vi "AlGaAs_SL_v07.vi"(2 "Debug Mode":bool, 3 "Elapsed Time(s)":dbl, 4 "State":enum16{"Edit", "Start", "Run", "End", "Idle"}(ring), 5 "Argument List In":string[](array[string])) -> (0 "Status Out":string, 1 "Argument List Out":string[](array[string]))   [LabVIEW 2011]
panel:
  out "tTotal(s) 2":dbl
  out "is_OK":bool
  out "tTotal(s)":dbl
  out "Do wait 2":bool
  out "Do wait 1":bool
  in  "Tab Control":enum32{"Step 1", "Step 2"}(tab)
  in  "run Ga 1":bool caption="run Ga"
  in  "run Al 1":bool=TRUE caption="run Al"
  in  "Al flow 1":dbl caption="Al flow(0-100sccm)" format="%.1f"
  in  "tFlow 1":dbl caption="tFlow(s)"
  in  "tWait(s) 1":dbl caption="tWait(s)"
  in  "Ga flow 1":dbl caption="Ga flow(0-10sccm)" format="%.3f"
  in  "fGa dilution 1":dbl caption="fGa dilution(>=1)"
  in  "run Ga 2":bool=TRUE caption="run Ga"
  in  "run Al 2":bool caption="run Al"
  in  "fGa 2":dbl caption="fGa dilution(>=1)"
  in  "Al flow 2":dbl caption="Al flow (0-100sccm)" format="%.1f"
  in  "Ga flow 2":dbl caption="Ga flow (0-10sccm)" format="%.3f"
  in  "tFlow 2":dbl caption="tFlow(s)"
  in  "tWait 2":dbl caption="tWait(s)"
  out "tphase(s)":dbl[](array[numeric])
  out "nstep":dbl
  out "phase":i32
  out "is_done":bool
  in  "nPeriods":dbl
  out "tPeriod(s)":dbl
  in  "Cancel":bool
  in  "OK":bool
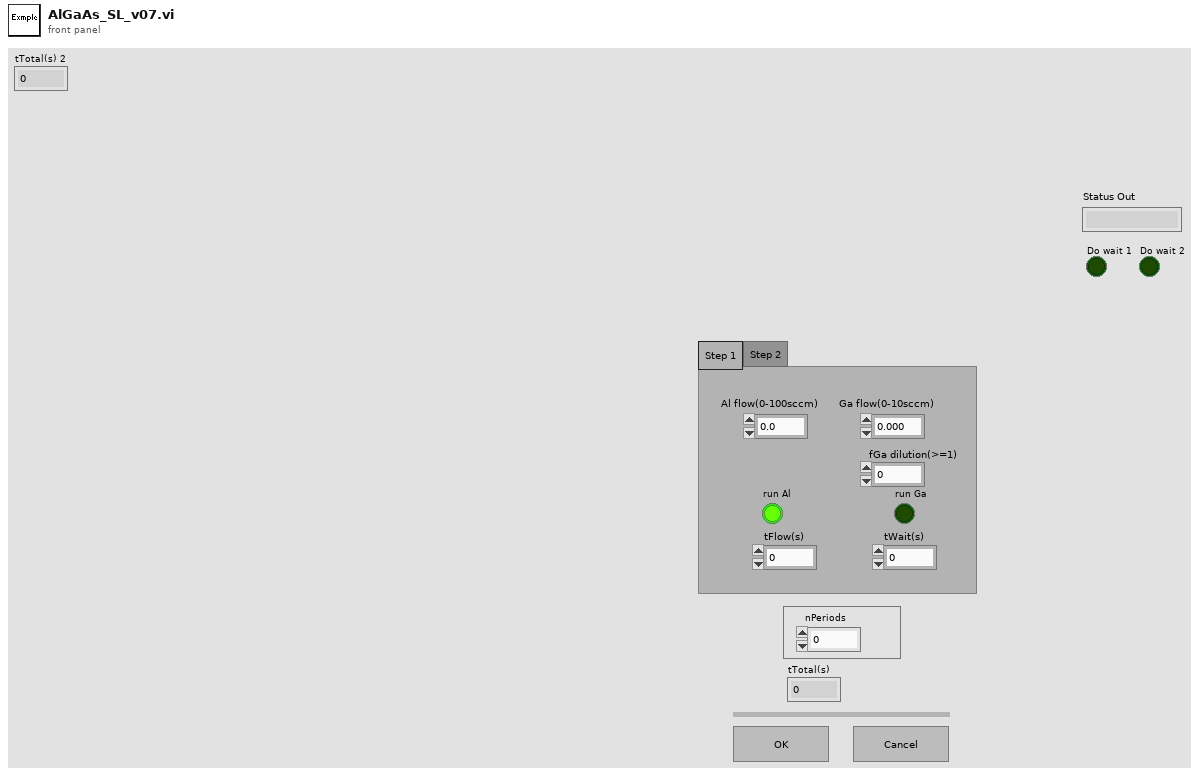
[diagram p1: front panel]
types:
  T1 = enum16{"Discrete", "Continuous", "Instantaneous"}
  T2 = enum32{"Invalid", "Default", "Floating", "Floating/Auto-Hide", "Modal"}
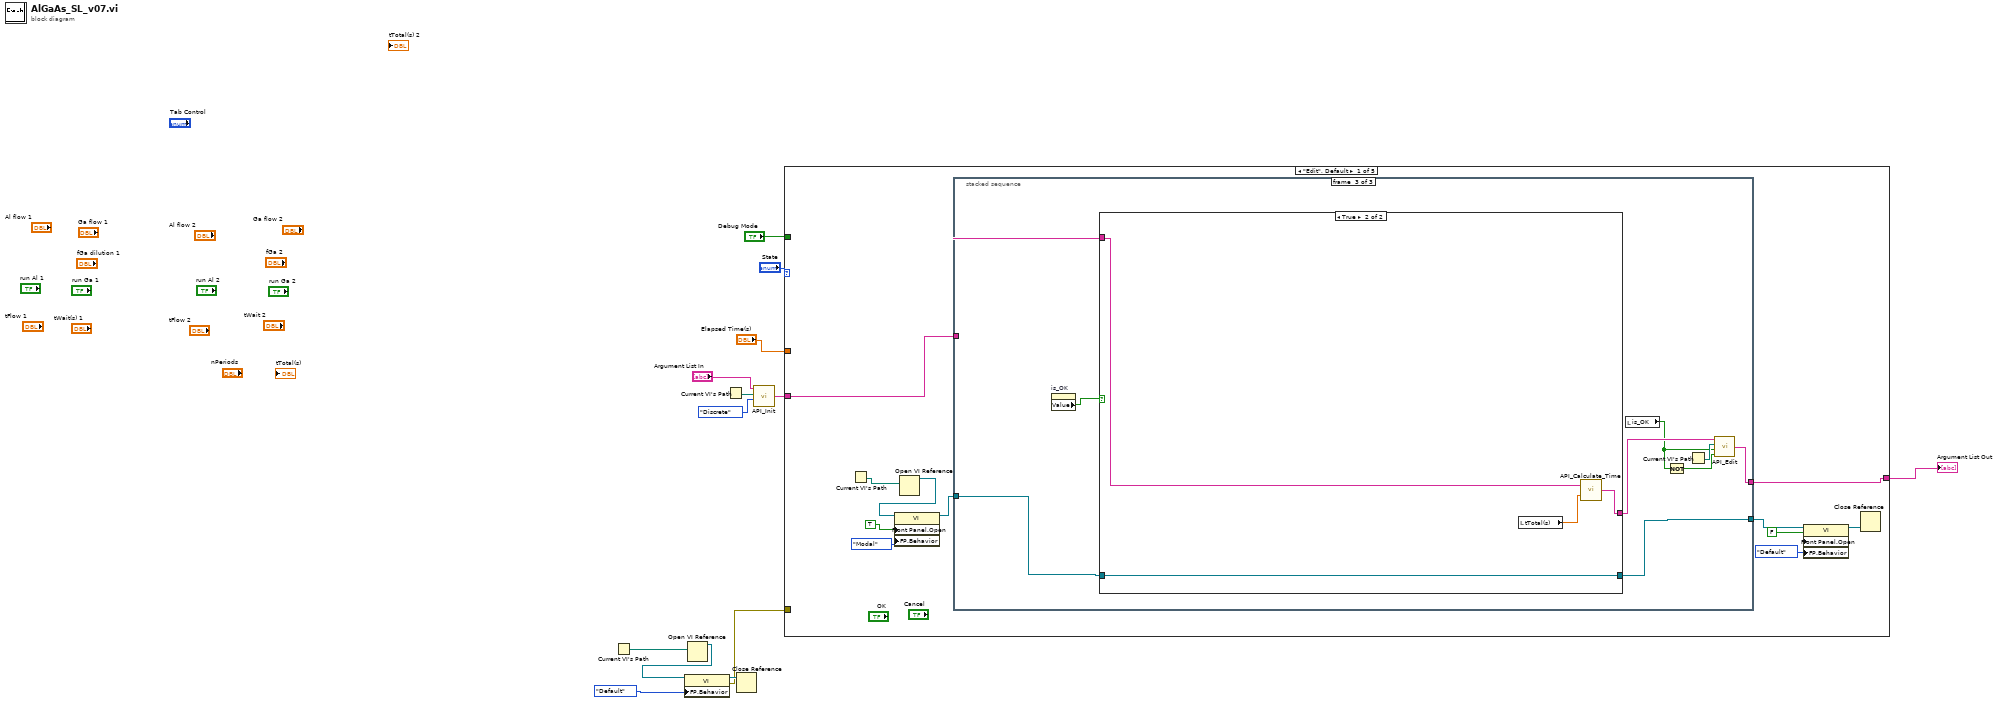
[diagram p0: block diagram]
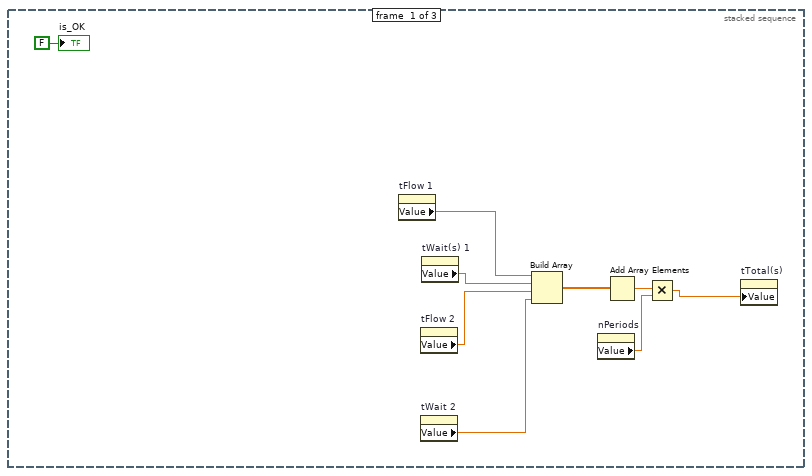
[diagram p2: hidden frame]
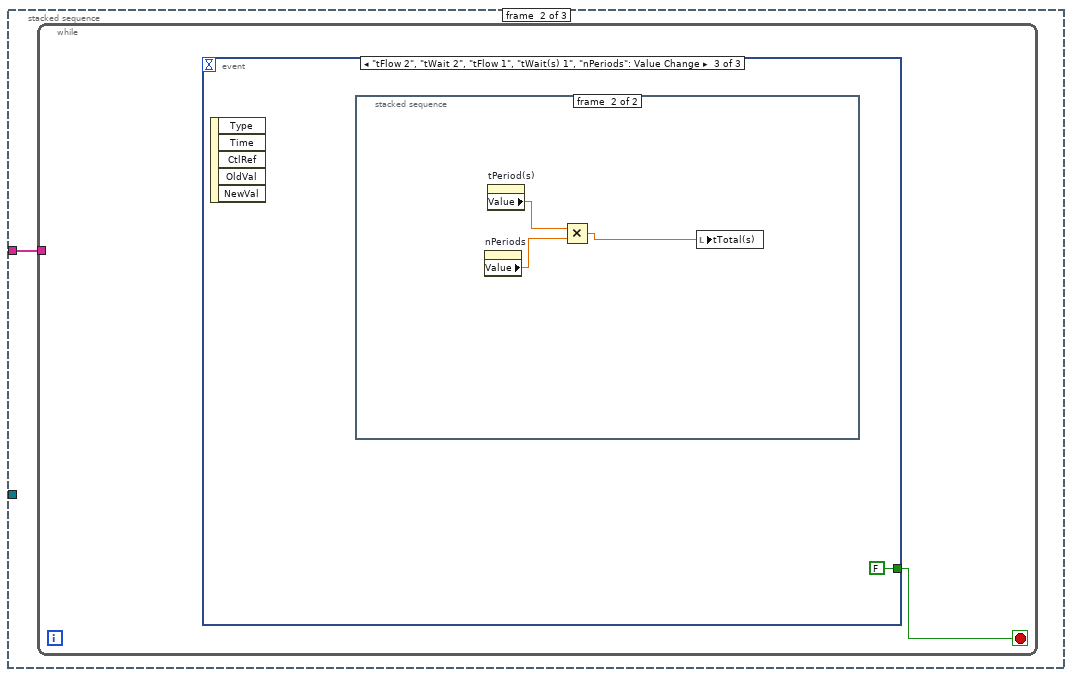
[diagram p3: hidden frame]
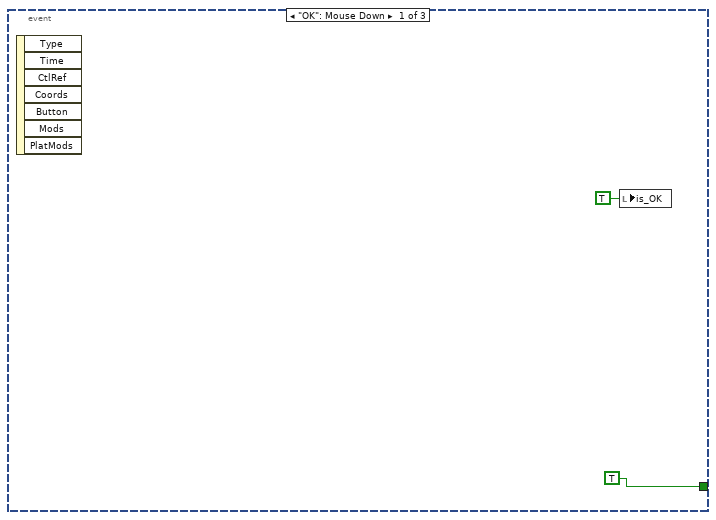
[diagram p4: hidden frame]
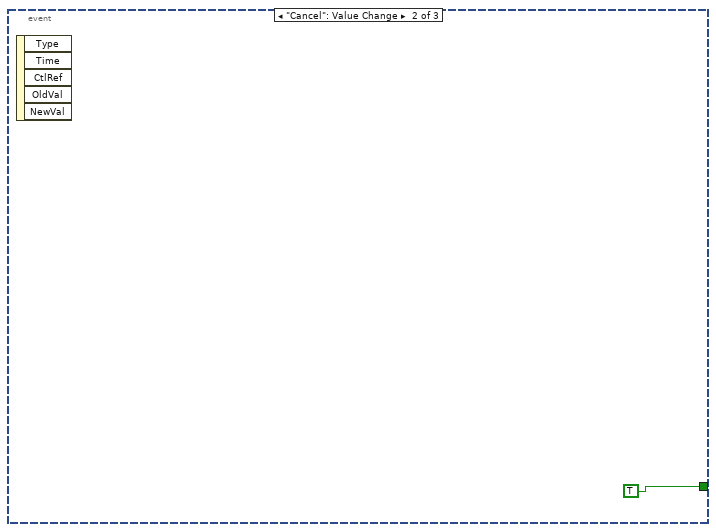
[diagram p5: hidden frame]
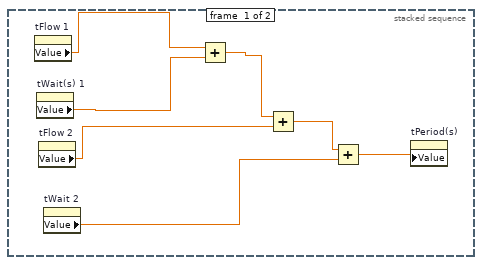
[diagram p6: hidden frame]
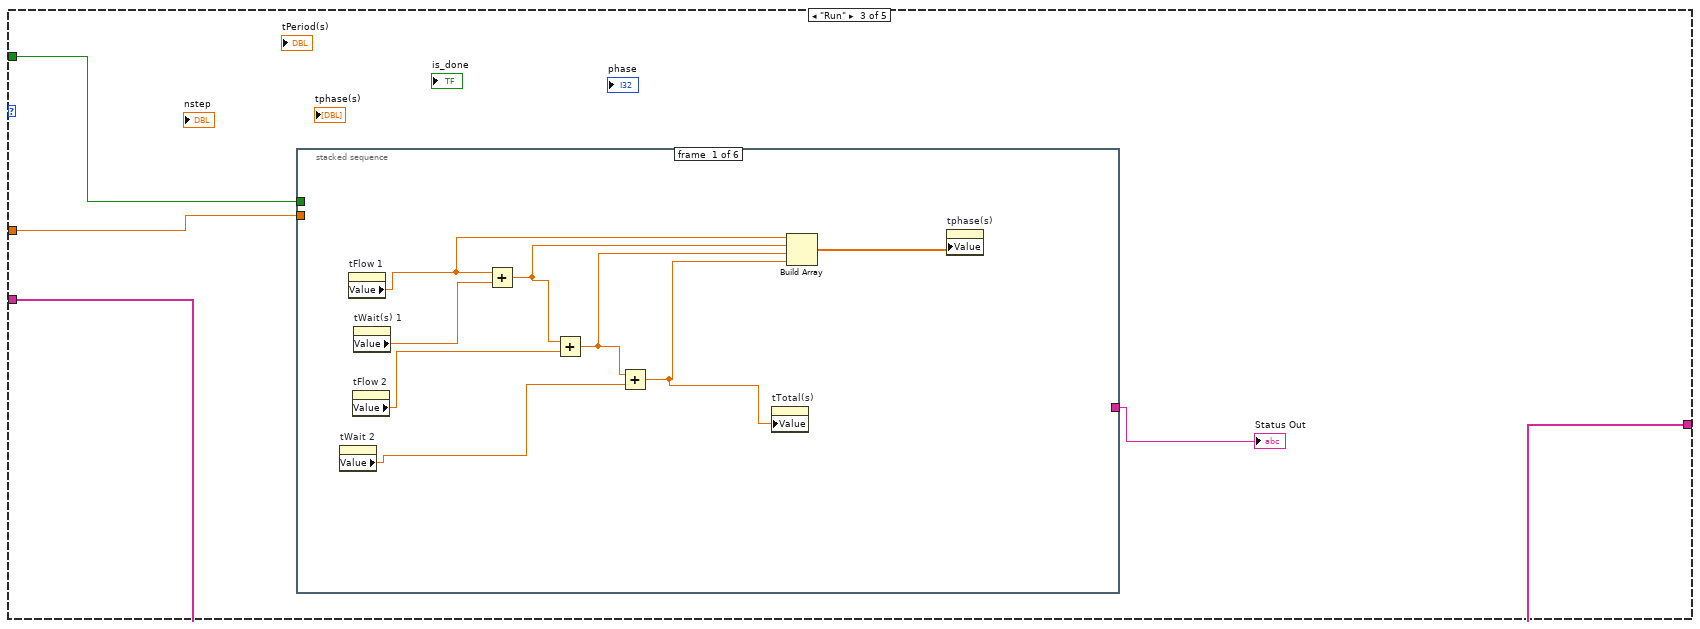
[diagram p9: hidden frame]
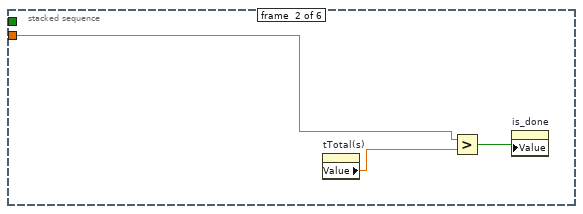
[diagram p10: hidden frame]
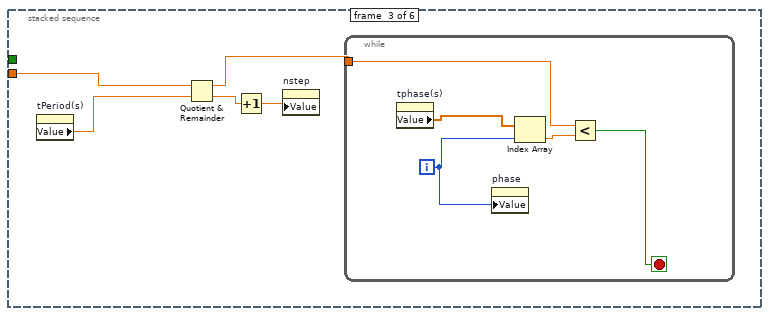
[diagram p11: hidden frame]
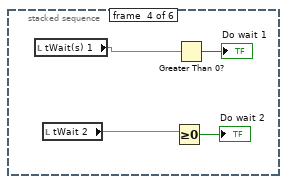
[diagram p12: hidden frame]
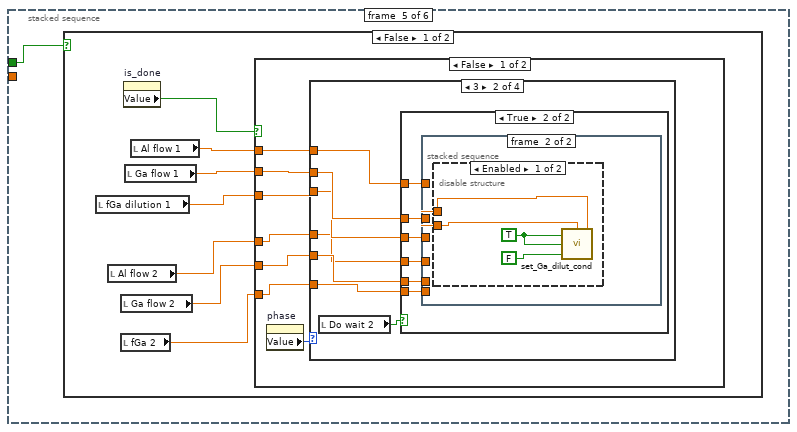
[diagram p13: hidden frame]
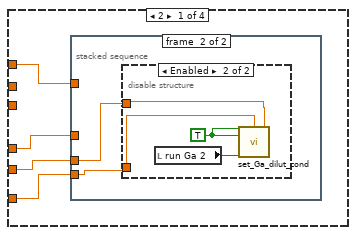
[diagram p14: hidden frame]
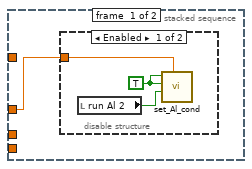
[diagram p15: hidden frame]
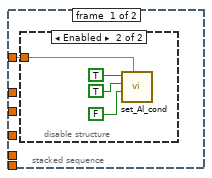
[diagram p19: hidden frame]
diagram:
  n1 = Current VI's Path() -> (path=w9:path)
  n2 = Open VI Reference(vi path=w9) -> (vi reference=w8:refnum<vi>)  [unwired: 1 in, 5 out]
  n3 = property class="VI"(reference=w8, "FP.Behavior"=T2."Default" ("Front Panel Window:Behavior")) -> (reference out=w6:refnum<vi>, error out=w5:errorcluster)  [unwired: 1 in]
  n4 = Current VI's Path() -> (path=w4:path)
  n5 = Close Reference(reference=w6) -> ()  [unwired: 1 in, 1 out]
  n6 = call "API_Init.vi"("API Mode"=T1."Discrete", "VI Path"=w4, "Argument List In"="Argument List In") -> ("Argument List Out"=w1:string[])  [unwired: 1 in]
  n7 = case shown="\"Edit\", Default" "State" {
    tunnel: "Debug Mode" -> [_ _ w68 _ _]
    tunnel: "Elapsed Time(s)" -> [_ _ w69 _ _]
    tunnel: w1 -> [w14 w65 w66 w242 w243]
    tunnel: [w21 w65 w66 w242 w243] -> w10
    tunnel: w5 -> [_ _ _ _ _]
    frame "Edit", Default {
      n8 = Current VI's Path() -> (path=w19:path)
      n9 = Open VI Reference(vi path=w19) -> (vi reference=w18:refnum<vi>)  [unwired: 1 in, 5 out]
      n10 = property class="VI"(reference=w18, "Front Panel.Open"=TRUE ("Front Panel Window:Open"), "FP.Behavior"=T2."Modal" ("Front Panel Window:Behavior")) -> (reference out=w17:refnum<vi>)  [unwired: 1 in, 1 out]
      n11 = stacked-sequence {
        tunnel: w14 -> [_ w34 w58]
        tunnel: w17 -> [_ _ w56]
        tunnel: [_ _ w55] -> w22
        tunnel: [_ _ w52] -> w21
        frame #0 {
          n12 = property on="tFlow 1" class="DigNum (strict)"() -> ("Value"=w26:dbl)  [unwired: 2 in, 2 out]
          n13 = property on="tFlow 2" class="DigNum (strict)"() -> ("Value"=w28:dbl)  [unwired: 2 in, 2 out]
          n14 = property on="tWait 2" class="DigNum (strict)"() -> ("Value"=w29:dbl)  [unwired: 2 in, 2 out]
          n15 = property on="tWait(s) 1" class="DigNum (strict)"() -> ("Value"=w27:dbl)  [unwired: 2 in, 2 out]
          n16 = Build Array(w26, w27, w28, w29) -> (w30:dbl[])
          n17 = property on="nPeriods" class="DigNum (strict)"() -> ("Value"=w32:dbl)  [unwired: 2 in, 2 out]
          n18 = Add Array Elements(numeric array=w30) -> (sum=w31:dbl)
          n19 = Multiply(x=w31, y=w32) -> (x*y=w33:dbl)
          n20 = property on="tTotal(s)" class="DigNum (strict)"("Value"=w33) -> ()  [unwired: 2 in, 2 out]
          "is_OK" <- FALSE ("is_OK")
        }
        frame #1 {
          n21 = while {
            tunnel: w34 -> [_]
            stop <- w35 stop-if-true
            n22 = event shown="[2] \"tFlow 2\", \"tWait 2\", \"tFlow 1\", \"tWait(s) 1\", \"nPeriods\": Value Change" {
              selector: _ -> [_ _ _]
              dyn-events: _ -> [_ _ _]
              timeout: _ -> [_ _ _]
              tunnel: [TRUE ("done_editing") TRUE ("done_editing") FALSE ("done_editing")] -> w35
              event "OK": Mouse Down {
                n23 = event-data() -> ()  [unwired: 1 in, 7 out]
                n24 = local write "is_OK"(TRUE ("is_OK")) -> ()
              }
              event "Cancel": Value Change {
                n25 = event-data() -> ()  [unwired: 1 in, 5 out]
              }
              event "tFlow 2", "tWait 2", "tFlow 1", "tWait(s) 1", "nPeriods": Value Change {
                n26 = event-data() -> ()  [unwired: 1 in, 5 out]
                n27 = stacked-sequence {
                  frame #0 {
                    n28 = property on="tFlow 1" class="DigNum (strict)"() -> ("Value"=w43:dbl)  [unwired: 2 in, 2 out]
                    n29 = property on="tWait(s) 1" class="DigNum (strict)"() -> ("Value"=w44:dbl)  [unwired: 2 in, 2 out]
                    n30 = property on="tFlow 2" class="DigNum (strict)"() -> ("Value"=w45:dbl)  [unwired: 2 in, 2 out]
                    n31 = property on="tWait 2" class="DigNum (strict)"() -> ("Value"=w40:dbl)  [unwired: 2 in, 2 out]
                    n32 = Add(x=w43, y=w44) -> (x+y=w42:dbl)
                    n33 = Add(x=w42, y=w45) -> (x+y=w41:dbl)
                    n34 = Add(x=w41, y=w40) -> (x+y=w46:dbl)
                    n35 = property on="tPeriod(s)" class="DigNum (strict)"("Value"=w46) -> ()  [unwired: 2 in, 2 out]
                  }
                  frame #1 {
                    n36 = property on="nPeriods" class="DigNum (strict)"() -> ("Value"=w48:dbl)  [unwired: 2 in, 2 out]
                    n37 = property on="tPeriod(s)" class="DigNum (strict)"() -> ("Value"=w49:dbl)  [unwired: 2 in, 2 out]
                    n38 = Multiply(x=w49, y=w48) -> (x*y=w47:dbl)
                    n39 = local write "tTotal(s)"(w47) -> ()
                  }
                }
              }
            }
          }
        }
        frame #2 {
          n40 = property on="is_OK" class="Bool (strict)"() -> ("Value"=w57:bool)  [unwired: 2 in, 2 out]
          n41 = case shown="True" w57 {
            tunnel: w58 -> [w60 w61]
            tunnel: [w60 w63] -> w53
            tunnel: w56 -> [w59 w64]
            tunnel: [w59 w64] -> w55
            frame False {
            }
            frame True {
              n42 = local read "tTotal(s)"() -> (w62:dbl)
              n43 = call "API_Calculate_Time.vi"("Time"=w62, "Argument List In"=w61) -> ("Argument List Out"=w63:string[])
            }
          }
          n44 = local read "is_OK"() -> (w51:bool)
          n45 = Not(x=w51) -> (.not. x?=w50:bool)
          n46 = Current VI's Path() -> (path=w54:path)
          n47 = call "API_Edit.vi"("Cancel"=w50, "OK"=w51, "VI Path"=w54, "Argument List In"=w53) -> ("Argument List Out"=w52:string[])
        }
      }
      n48 = property class="VI"(reference=w22, "Front Panel.Open"=FALSE ("Front Panel Window:Open"), "FP.Behavior"=T2."Default" ("Front Panel Window:Behavior")) -> (reference out=w23:refnum<vi>)  [unwired: 1 in, 1 out]
      n49 = Close Reference(reference=w23) -> ()  [unwired: 1 in, 1 out]
    }
    frame "Start" {
    }
    frame "Run" {
      n50 = stacked-sequence {
        tunnel: w69 -> [_ w78 w85 _ _ _]
        tunnel: w68 -> [_ _ _ _ w95 _]
        tunnel: [_ _ _ _ _ w194] -> w67
        frame #0 {
          n51 = property on="tWait 2" class="DigNum (strict)"() -> ("Value"=w71:dbl)  [unwired: 2 in, 2 out]
          n52 = property on="tFlow 1" class="DigNum (strict)"() -> ("Value"=w74:dbl)  [unwired: 2 in, 2 out]
          n53 = property on="tFlow 2" class="DigNum (strict)"() -> ("Value"=w72:dbl)  [unwired: 2 in, 2 out]
          n54 = property on="tWait(s) 1" class="DigNum (strict)"() -> ("Value"=w73:dbl)  [unwired: 2 in, 2 out]
          n55 = Add(x=w74, y=w73) -> (x+y=w77:dbl)
          n56 = Add(x=w77, y=w72) -> (x+y=w76:dbl)
          n57 = Add(x=w76, y=w71) -> (x+y=w70:dbl)
          n58 = property on="tTotal(s)" class="DigNum (strict)"("Value"=w70) -> ()  [unwired: 2 in, 2 out]
          n59 = Build Array(w74, w77, w76, w70) -> (w75:dbl[])
          n60 = property on="tphase(s)" class="Arr (strict)"("Value"=w75) -> ()  [unwired: 2 in, 2 out]
        }
        frame #1 {
          n61 = property on="tTotal(s)" class="DigNum (strict)"() -> ("Value"=w79:dbl)  [unwired: 2 in, 2 out]
          n62 = Greater?(x=w78, y=w79) -> (0:w80:bool)
          n63 = property on="is_done" class="Bool (strict)"("Value"=w80) -> ()  [unwired: 2 in, 2 out]
        }
        frame #2 {
          n64 = property on="tPeriod(s)" class="DigNum (strict)"() -> ("Value"=w84:dbl)  [unwired: 2 in, 2 out]
          n65 = Quotient & Remainder(x=w85, y=w84) -> (x-y*floor(x/y)=w83:dbl, floor(x/y)=w82:dbl)
          n66 = Increment(x=w82) -> (x+1=w81:dbl)
          n67 = property on="nstep" class="DigNum (strict)"("Value"=w81) -> ()  [unwired: 2 in, 2 out]
          n68 = while {
            tunnel: w83 -> [w89]
            i -> [w87]
            stop <- w86 stop-if-true
            n69 = property on="tphase(s)" class="Arr (strict)"() -> ("Value"=w90:dbl[])  [unwired: 2 in, 2 out]
            n70 = property on="phase" class="DigNum (strict)"("Value"=w87) -> ()  [unwired: 2 in, 2 out]
            n71 = Index Array(array=w90, index=w87) -> (element=w88:dbl)
            n72 = Less?(x=w89, y=w88) -> (x < y?=w86:bool)
          }
        }
        frame #3 {
          n73 = local read "tWait(s) 1"() -> (w94:dbl)
          n74 = local read "tWait 2"() -> (w92:dbl)
          n75 = Greater Or Equal To 0?(x=w92) -> (x >= 0?=→"Do wait 2":bool)
          n76 = Greater Than 0?(x=w94) -> (x > 0?=→"Do wait 1":bool)
        }
        frame #4 {
          n77 = case shown="False" w95 {
            frame False {
              n78 = local read "fGa dilution 1"() -> (w98:dbl)
              n79 = local read "Al flow 2"() -> (w97:dbl)
              n80 = local read "Ga flow 2"() -> (w102:dbl)
              n81 = local read "fGa 2"() -> (w96:dbl)
              n82 = property on="is_done" class="Bool (strict)"() -> ("Value"=w100:bool)  [unwired: 2 in, 2 out]
              n83 = local read "Ga flow 1"() -> (w99:dbl)
              n84 = local read "Al flow 1"() -> (w101:dbl)
              n85 = case shown="False" w100 {
                tunnel: w102 -> [w109 w184]
                tunnel: w101 -> [w108 w185]
                tunnel: w99 -> [w106 _]
                tunnel: w98 -> [w105 _]
                tunnel: w97 -> [w104 _]
                tunnel: w96 -> [w103 _]
                frame False {
                  n86 = property on="phase" class="DigNum (strict)"() -> ("Value"=w107:i32)  [unwired: 2 in, 2 out]
                  n87 = case shown="3" w107 {
                    tunnel: w108 -> [w113 w130 w150 w167]
                    tunnel: w109 -> [w112 w129 _ w163]
                    tunnel: w106 -> [_ w128 w149 w165]
                    tunnel: w105 -> [_ w127 w148 w166]
                    tunnel: w104 -> [w110 w126 _ w164]
                    tunnel: w103 -> [w111 w125 _ w162]
                    frame 2 {
                      n88 = stacked-sequence {
                        tunnel: w113 -> [_ _]
                        tunnel: w112 -> [_ w119]
                        tunnel: w111 -> [_ w118]
                        tunnel: w110 -> [w114 _]
                        frame #0 {
                          n89 = disable-structure shown="Enabled" {
                            disable-tunnel: w114 -> [w117 _]
                            frame Enabled {
                              w116 = TRUE ("Ga Active")
                              n90 = local read "run Al 2"() -> (w115:bool)
                              n91 = call "set_Al_cond.vi"("Aluminum Flow"=w117, "Al Run"=w115, "Al Bubbler"=w116, "Al Active"=w116) -> ()  [unwired: 6 in]
                            }
                            frame Disabled {
                            }
                          }
                        }
                        frame #1 {
                          n92 = disable-structure shown="Enabled" {
                            disable-tunnel: w119 -> [_ w123]
                            disable-tunnel: w118 -> [_ w122]
                            frame Disabled {
                            }
                            frame Enabled {
                              w121 = TRUE ("Ga Active")
                              n93 = local read "run Ga 2"() -> (w120:bool)
                              n94 = call "set_Ga_dilut_cond.vi"("Ga flow (0-10 sccm)"=w123, "fDilution"=w122, "Run"=w120, "Bubbler In"=w121, "Active"=w121) -> ()
                            }
                          }
                        }
                      }
                    }
                    frame 3 {
                      n95 = local read "Do wait 2"() -> (w124:bool)
                      n96 = case shown="True" w124 {
                        tunnel: w130 -> [_ w136]
                        tunnel: w129 -> [_ w135]
                        tunnel: w128 -> [_ w134]
                        tunnel: w127 -> [_ w133]
                        tunnel: w126 -> [_ w132]
                        tunnel: w125 -> [_ w131]
                        frame False {
                        }
                        frame True {
                          n97 = stacked-sequence {
                            tunnel: w136 -> [w137 _]
                            tunnel: w135 -> [_ _]
                            tunnel: w134 -> [_ w143]
                            tunnel: w133 -> [_ w142]
                            tunnel: w132 -> [_ _]
                            tunnel: w131 -> [_ _]
                            frame #0 {
                              n98 = disable-structure shown="Enabled" {
                                disable-tunnel: w137 -> [_ w138]
                                frame Disabled {
                                }
                                frame Enabled {
                                n99 = call "set_Al_cond.vi"("Aluminum Flow"=w138, "Al Run"=FALSE, "Al Bubbler"=TRUE, "Al Active"=TRUE) -> ()  [unwired: 6 in]
                                }
                              }
                            }
                            frame #1 {
                              n100 = disable-structure shown="Enabled" {
                                disable-tunnel: w143 -> [w147 _]
                                disable-tunnel: w142 -> [w146 _]
                                frame Enabled {
                                w145 = TRUE ("Ga Active")
                                n101 = call "set_Ga_dilut_cond.vi"("Ga flow (0-10 sccm)"=w147, "fDilution"=w146, "Run"=FALSE ("Ga Run"), "Bubbler In"=w145, "Active"=w145) -> ()
                                }
                                frame Disabled {
                                }
                              }
                            }
                          }
                        }
                      }
                    }
                    frame 0, Default {
                      n102 = stacked-sequence {
                        tunnel: w150 -> [w151 _]
                        tunnel: w149 -> [_ w156]
                        tunnel: w148 -> [_ w155]
                        frame #0 {
                          n103 = disable-structure shown="Enabled" {
                            disable-tunnel: w151 -> [_ w154]
                            frame Disabled {
                            }
                            frame Enabled {
                              w153 = TRUE ("Al Active")
                              n104 = local read "run Al 1"() -> (w152:bool)
                              n105 = call "set_Al_cond.vi"("Aluminum Flow"=w154, "Al Run"=w152, "Al Bubbler"=w153, "Al Active"=w153) -> ()  [unwired: 6 in]
                            }
                          }
                        }
                        frame #1 {
                          n106 = disable-structure shown="Enabled" {
                            disable-tunnel: w156 -> [w160 _]
                            disable-tunnel: w155 -> [w159 _]
                            frame Enabled {
                              w158 = TRUE ("Ga Active")
                              n107 = local read "run Ga 1"() -> (w157:bool)
                              n108 = call "set_Ga_dilut_cond.vi"("Ga flow (0-10 sccm)"=w160, "fDilution"=w159, "Run"=w157, "Bubbler In"=w158, "Active"=w158) -> ()
                            }
                            frame Disabled {
                            }
                          }
                        }
                      }
                    }
                    frame 1 {
                      n109 = local read "Do wait 1"() -> (w161:bool)
                      n110 = case shown="True" w161 {
                        tunnel: w167 -> [_ w173]
                        tunnel: w166 -> [_ w172]
                        tunnel: w165 -> [_ w171]
                        tunnel: w164 -> [_ w170]
                        tunnel: w163 -> [_ w169]
                        tunnel: w162 -> [_ w168]
                        frame False {
                        }
                        frame True {
                          n111 = stacked-sequence {
                            tunnel: w173 -> [_ _]
                            tunnel: w172 -> [_ _]
                            tunnel: w171 -> [_ _]
                            tunnel: w170 -> [w174 _]
                            tunnel: w169 -> [_ w178]
                            tunnel: w168 -> [_ w179]
                            frame #0 {
                              n112 = disable-structure shown="Enabled" {
                                disable-tunnel: w174 -> [_ w175]
                                frame Disabled {
                                }
                                frame Enabled {
                                w176 = TRUE ("Al Bubbler")
                                n113 = call "set_Al_cond.vi"("Aluminum Flow"=w175, "Al Run"=FALSE, "Al Bubbler"=w176, "Al Active"=w176) -> ()  [unwired: 6 in]
                                }
                              }
                            }
                            frame #1 {
                              n114 = disable-structure shown="Enabled" {
                                disable-tunnel: w178 -> [w181 _]
                                disable-tunnel: w179 -> [w180 _]
                                frame Enabled {
                                w182 = TRUE ("Ga Active")
                                n115 = call "set_Ga_dilut_cond.vi"("Ga flow (0-10 sccm)"=w181, "fDilution"=w180, "Run"=FALSE ("Ga Run"), "Bubbler In"=w182, "Active"=w182) -> ()
                                }
                                frame Disabled {
                                }
                              }
                            }
                          }
                        }
                      }
                    }
                  }
                }
                frame True {
                  n116 = stacked-sequence {
                    tunnel: w185 -> [w186 _]
                    tunnel: w184 -> [_ w190]
                    frame #0 {
                      n117 = disable-structure shown="Enabled" {
                        disable-tunnel: w186 -> [_ w189]
                        frame Disabled {
                        }
                        frame Enabled {
                          w188 = TRUE ("Al Active")
                          n118 = call "set_Al.vi"("Aluminum Flow"=w189, "Al Run"=FALSE, "Al Bubbler"=w188, "Al Active"=w188) -> ()  [unwired: 6 in]
                        }
                      }
                    }
                    frame #1 {
                      n119 = disable-structure shown="Enabled" {
                        disable-tunnel: w190 -> [w191 _]
                        frame Enabled {
                          w192 = TRUE ("Ga Active")
                          n120 = call "set_Ga.vi"("Ga Active"=w192, "Ga Flow 1"=w191, "Ga Bubbler"=w192, "Ga Run"=FALSE) -> ()  [unwired: 4 in, 8 out]
                        }
                        frame Disabled {
                        }
                      }
                    }
                  }
                }
              }
            }
            frame True {
            }
          }
        }
        frame #5 {
          n121 = property on="is_done" class="Bool (strict)"() -> ("Value"=w195:bool)  [unwired: 2 in, 2 out]
          n122 = case shown="False" w195 {
            tunnel: [w204 w241] -> w194
            frame False {
              w198 = ", " ("string")
              n123 = property on="phase" class="DigNum (strict)"() -> ("Value"=w197:i32)  [unwired: 2 in, 2 out]
              n124 = Increment(x=w197) -> (x+1=w196:i32)
              n125 = Format Into String(format string="%2.0f", w196) -> (resulting string=w202:string)  [unwired: 2 in, 1 out]
              n126 = case shown="3" w197 {
                tunnel: [w212 "wait (after 2)" w223 "wait (after 1)"] -> w199
                frame 2 {
                  n127 = local read "Ga flow 2"() -> (w214:dbl)
                  n128 = local read "Al flow 2"() -> (w215:dbl)
                  n129 = Format Into String(format string="%4.1f", w215) -> (resulting string=w218:string)  [unwired: 2 in, 1 out]
                  n130 = Format Into String(format string="%4.1f", w214) -> (resulting string=w221:string)  [unwired: 2 in, 1 out]
                  n131 = Concatenate Strings("Al(" ("string"), w218, "sccm)" ("string")) -> (w213:string)
                  n132 = Concatenate Strings(w213, "Ga(" ("string"), w221, "sccm)" ("string")) -> (w212:string)
                }
                frame 3 {
                }
                frame 0, Default {
                  n133 = local read "Al flow 1"() -> (w230:dbl)
                  n134 = local read "Ga flow 1"() -> (w229:dbl)
                  n135 = Format Into String(format string="%4.1f", w230) -> (resulting string=w232:string)  [unwired: 2 in, 1 out]
                  n136 = Format Into String(format string="%4.1f", w229) -> (resulting string=w225:string)  [unwired: 2 in, 1 out]
                  n137 = Concatenate Strings("Al(" ("string"), w232, "sccm)" ("string")) -> (w224:string)
                  n138 = Concatenate Strings(w224, "Ga(" ("string"), w225, "sccm)" ("string")) -> (w223:string)
                }
                frame 1 {
                }
              }
              n139 = Concatenate Strings("Phase " ("string"), w202) -> (w200:string)
              n140 = property on="nstep" class="DigNum (strict)"() -> ("Value"=w209:dbl)  [unwired: 2 in, 2 out]
              n141 = Format Into String(format string="%3.0f", w209) -> (resulting string=w206:string)  [unwired: 2 in, 1 out]
              n142 = Concatenate Strings("Period " ("string"), w206) -> (w205:string)
              n143 = Concatenate Strings(w205, w198, w200, w198, w199) -> (w204:string)
            }
            frame True {
              n144 = property on="nPeriods" class="DigNum (strict)"() -> ("Value"=w236:dbl)  [unwired: 2 in, 2 out]
              n145 = Format Into String(format string="%3.0f", w236) -> (resulting string=w237:string)  [unwired: 2 in, 1 out]
              n146 = Concatenate Strings("done after", w237, " periods" ("string")) -> (w241:string)
            }
          }
        }
      }
      "Status Out" <- w67
    }
    frame "End" {
    }
    frame "Idle" {
    }
  }
  "Argument List Out" <- w10
